vi "Save Output Settings to CSV.vi"(0 "time stamp":timestamp, 1 "Event Name":cluster{"string":string, string}, 2 "Modulatin Depth Sweep Parameters":T1={"f (Hz)"=200.0, "Number of steps"=2, "Total time (s)"=2.0, "Amplitude (V)"=1.0, "depth_start (0.0 %)"=50.0, "Channel (1:Channel 1)"=2, "fc (Hz)"=2000.0, "DC Offset (V)"=0.0, "depth_end (0.0 %)"=50.0} {"depth_end (0.0 %)" min=0.0 max=120.0 format="%.1f"; "DC Offset (V)" min=-20.0 max=20.0 format="%#_13g"; "fc (Hz)" min=0.0; "Channel (1:Channel 1)" items=["Channel 1"=1, "Channel 2"=2]; "depth_start (0.0 %)" min=0.0 max=120.0 format="%.1f"; "Amplitude (V)" min=0.0 max=20.0 format="%#_13g"; "Total time (s)" min=0.0; "Number of steps" min=2; "f (Hz)" min=0.0}, 3 "File numbers":i32[](array[numeric]), 4 "File Parameters":cluster{"Path":path, "Recording Name":string}={"Path"=path "D:/data/Lucas/20210707_lucas_test_saving", "Recording Name"=""}, 5 "error in (no error)":errorcluster, 6 "Output Parameters":T6={"Signal Parameters"={"P2P Amplitude (V)"=3.0, "Frequency (Hz)"=100000.0, "DC Offset ( V)"=0.0, "Waveform Function (0: Sine)"=0}, "Modulation Parameters"={"Waveform"=0, "Frequency (Hz)"=1000.0, "Depth (%)"=0.0, "Type"=100}} {"Modulation Parameters"."Type" items=["Amplitude", "Frequency"]; "Modulation Parameters"."Depth (%)" min=0.0 max=100.0 format="%.1f"; "Modulation Parameters"."Waveform" items=["Sine", "Square", "Triangle", "UpRamp", "DnRamp", "Noise", "Arb"]; "Signal Parameters"."Waveform Function (0: Sine)" items=["Sine", "Square", "Triangle", "DC", "Pulse", "Arb"]; "Signal Parameters"."P2P Amplitude (V)" min=0.0 max=20.0}, 7 "DIO":T5, 8 "Frequency Sweep I Parameters":T4={"f_start (Hz)"=0.0, "f_end (Hz)"=0.0, "Number of steps"=2, "Total time (s)"=0.0, "fc (Hz)"=2000.0, "Modulation Depth (0.0 %)"=0.0, "Channel (1:Channel 1)"=1, "amp (V)"=1.0, "DC Offset (V)"=0.0} {"DC Offset (V)" min=-20.0 max=20.0 format="%#_13g"; "amp (V)" min=0.0 max=20.0 format="%#_13g"; "Channel (1:Channel 1)" items=["Channel 1"=1, "Channel 2"=2]; "Modulation Depth (0.0 %)" min=0.0 max=120.0 format="%.1f"; "fc (Hz)" min=0.0 format="%#_13g"; "Total time (s)" min=0.0; "Number of steps" min=2; "f_end (Hz)" min=0.0; "f_start (Hz)" min=0.0}, 9 "Channel output":bool, 10 "Frequency Sweep II Parameters":T3={"f (Hz)"=0.0, "Number of steps"=2, "Total time (s)"=0.0, "fc_start (Hz)"=2000.0, "Modulation Depth (0.0 %)"=0.0, "Channel (1:Channel 1)"=1, "fc_end (Hz)"=2000.0, "amp (V)"=1.0, "DC Offset (V)"=0.0} {"DC Offset (V)" min=-20.0 max=20.0 format="%#_13g"; "amp (V)" min=0.0 max=20.0 format="%#_13g"; "fc_end (Hz)" min=0.0 format="%#_13g"; "Channel (1:Channel 1)" items=["Channel 1"=1, "Channel 2"=2]; "Modulation Depth (0.0 %)" min=0.0 max=120.0 format="%.1f"; "fc_start (Hz)" min=0.0 format="%#_13g"; "Total time (s)" min=0.0; "Number of steps" min=2; "f (Hz)" min=0.0}, 11 "Channel Modulation":bool, 12 "Amplitude Sweep Parameters":T2={"f (Hz)"=0.0, "Number of steps"=2, "Total time (s)"=0.0, "amp_start (V)"=2000.0, "Modulation Depth (0.0 %)"=0.0, "Channel (1:Channel 1)"=2, "amp_end (V)"=2000.0, "fc (Hz)"=0.0, "DC Offset (V)"=0.0} {"DC Offset (V)" min=-20.0 max=20.0 format="%#_13g"; "fc (Hz)" min=0.0; "amp_end (V)" min=0.0 max=20.0 format="%#_13g"; "Channel (1:Channel 1)" items=["Channel 1"=1, "Channel 2"=2]; "Modulation Depth (0.0 %)" min=0.0 max=120.0 format="%.1f"; "amp_start (V)" min=0.0 max=20.0 format="%#_13g"; "Total time (s)" min=0.0; "Number of steps" min=2; "f (Hz)" min=0.0}, 13 "Threshold Value":u32, 16 "Precheck duration":u32, 17 "Scenario Duration":u32, 18 "Release Duration":u32) -> (14 "output filename":string, 19 "error out":errorcluster)   [LabVIEW 2024]
uses:
  Type Definitions/Channel Parameters.ctl
  Type Definitions/Modulation Types.ctl
  RT Core/Type Definitions/DIO_Cluster.ctl
  Type Definitions/Frequency_sweep_I Parameters.ctl
  Type Definitions/Frequency_sweep_II Parameters.ctl
  Type Definitions/Amplitude_sweep Parameters.ctl
  Type Definitions/Depth_sweep Parameters.ctl
  <vilib>/Utility/file.llb/Write Delimited Spreadsheet (string).vi
panel:
  out "Array":string[](array[string])
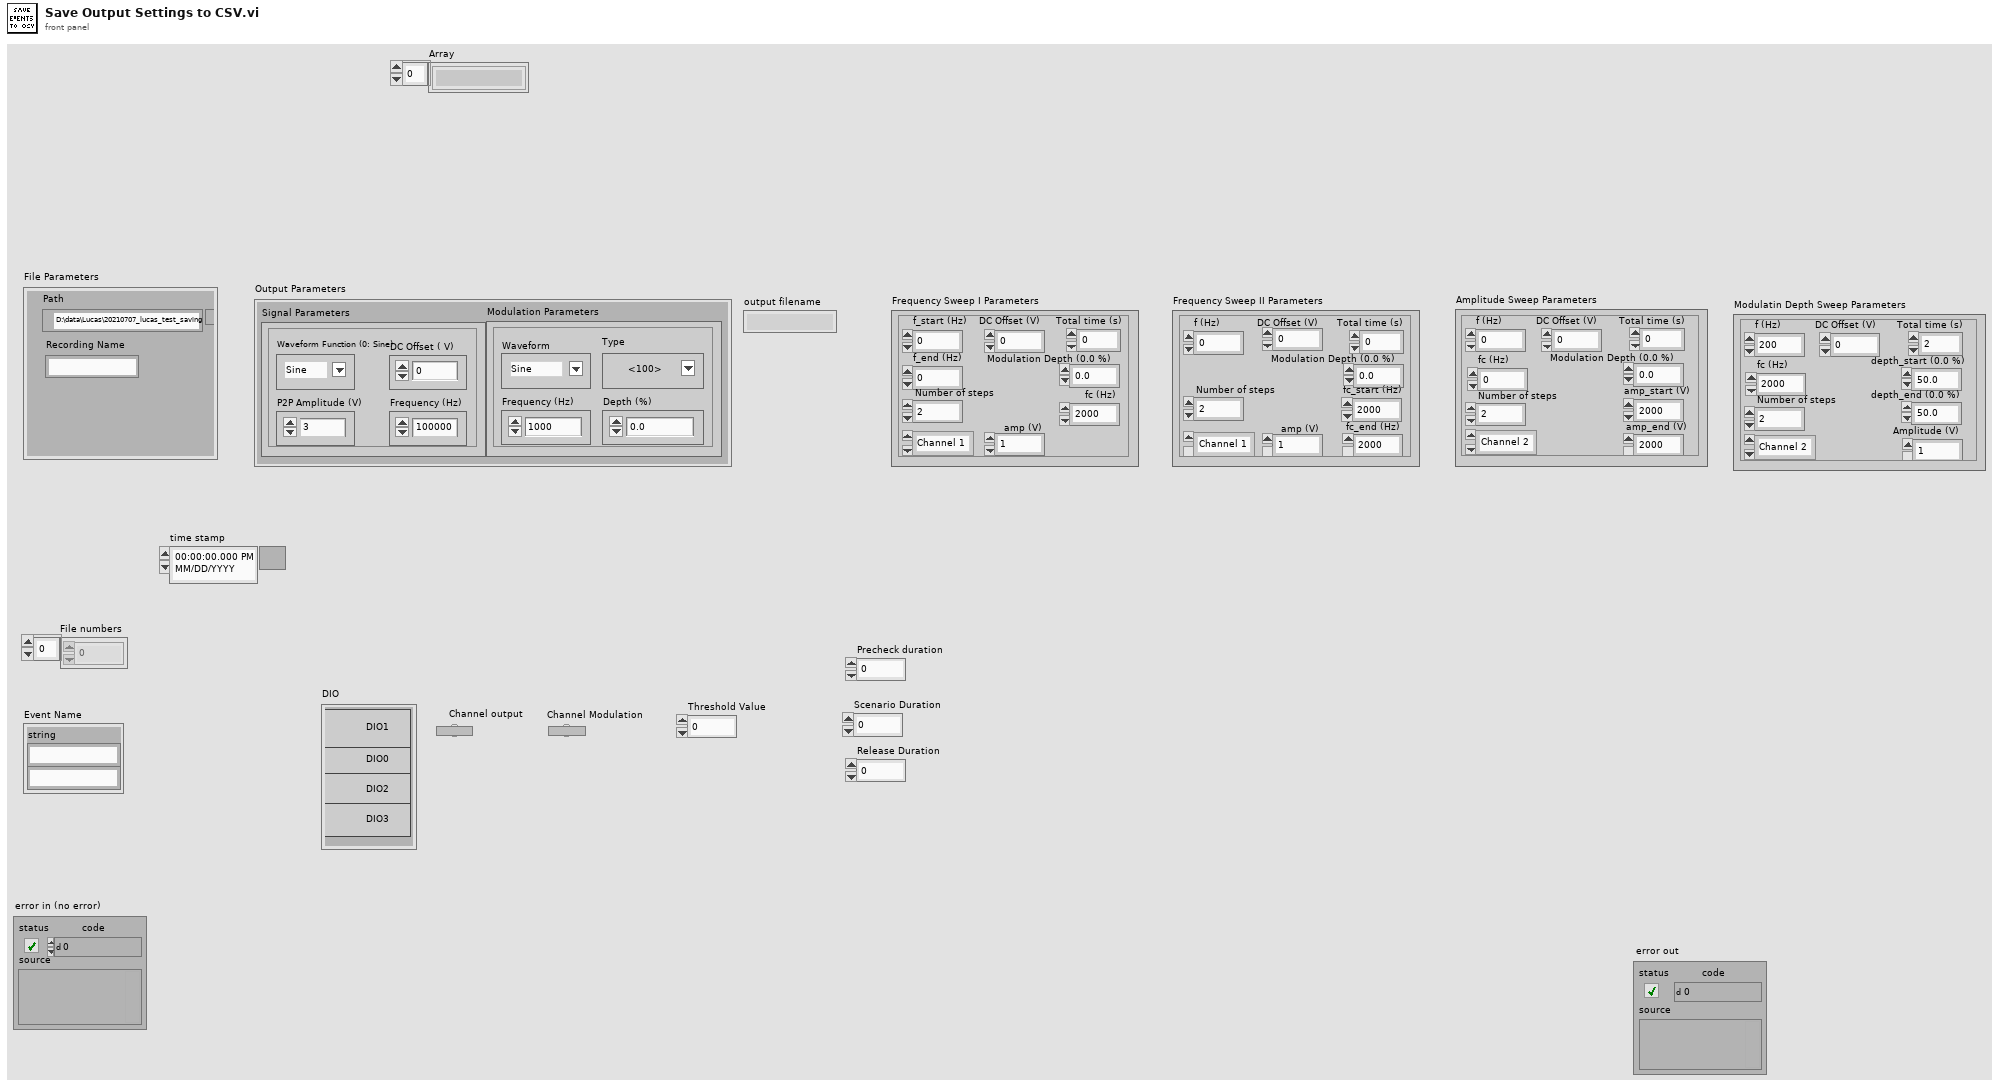
[diagram p1: front panel]
types:
  T1 = typedef "Depth_sweep Parameters.ctl" = cluster{"f (Hz)":dbl, "Number of steps":i32, "Total time (s)":dbl, "Amplitude (V)":dbl, "depth_start (0.0 %)":dbl, "Channel (1:Channel 1)":i32, "fc (Hz)":dbl, "DC Offset (V)":dbl, "depth_end (0.0 %)":dbl}
  T2 = typedef "Amplitude_sweep Parameters.ctl" = cluster{"f (Hz)":dbl, "Number of steps":i32, "Total time (s)":dbl, "amp_start (V)":dbl, "Modulation Depth (0.0 %)":dbl, "Channel (1:Channel 1)":i32, "amp_end (V)":dbl, "fc (Hz)":dbl, "DC Offset (V)":dbl}
  T3 = typedef "Frequency_sweep_II Parameters.ctl" = cluster{"f (Hz)":dbl, "Number of steps":i32, "Total time (s)":dbl, "fc_start (Hz)":dbl, "Modulation Depth (0.0 %)":dbl, "Channel (1:Channel 1)":i32, "fc_end (Hz)":dbl, "amp (V)":dbl, "DC Offset (V)":dbl}
  T4 = typedef "Frequency_sweep_I Parameters.ctl" = cluster{"f_start (Hz)":dbl, "f_end (Hz)":dbl, "Number of steps":i32, "Total time (s)":dbl, "fc (Hz)":dbl, "Modulation Depth (0.0 %)":dbl, "Channel (1:Channel 1)":i32, "amp (V)":dbl, "DC Offset (V)":dbl}
  T5 = typedef "DIO_Cluster.ctl" = cluster{"DIO0":bool, "DIO1":bool, "DIO2":bool, "DIO3":bool}
  T6 = typedef "Channel Parameters.ctl" = cluster{"Signal Parameters":cluster{"P2P Amplitude (V)":dbl, "Frequency (Hz)":dbl, "DC Offset ( V)":dbl, "Waveform Function (0: Sine)":u16}, "Modulation Parameters":cluster{"Waveform":u16, "Frequency (Hz)":dbl, "Depth (%)":dbl, "Type":T7}}
  T7 = typedef "Modulation Types.ctl" = u16
  T8 = cluster{"P2P Amplitude (V)":dbl, "Frequency (Hz)":dbl, "DC Offset ( V)":dbl, "Waveform Function (0: Sine)":u16}
  T9 = cluster{"Waveform":u16, "Frequency (Hz)":dbl, "Depth (%)":dbl, "Type":T7}
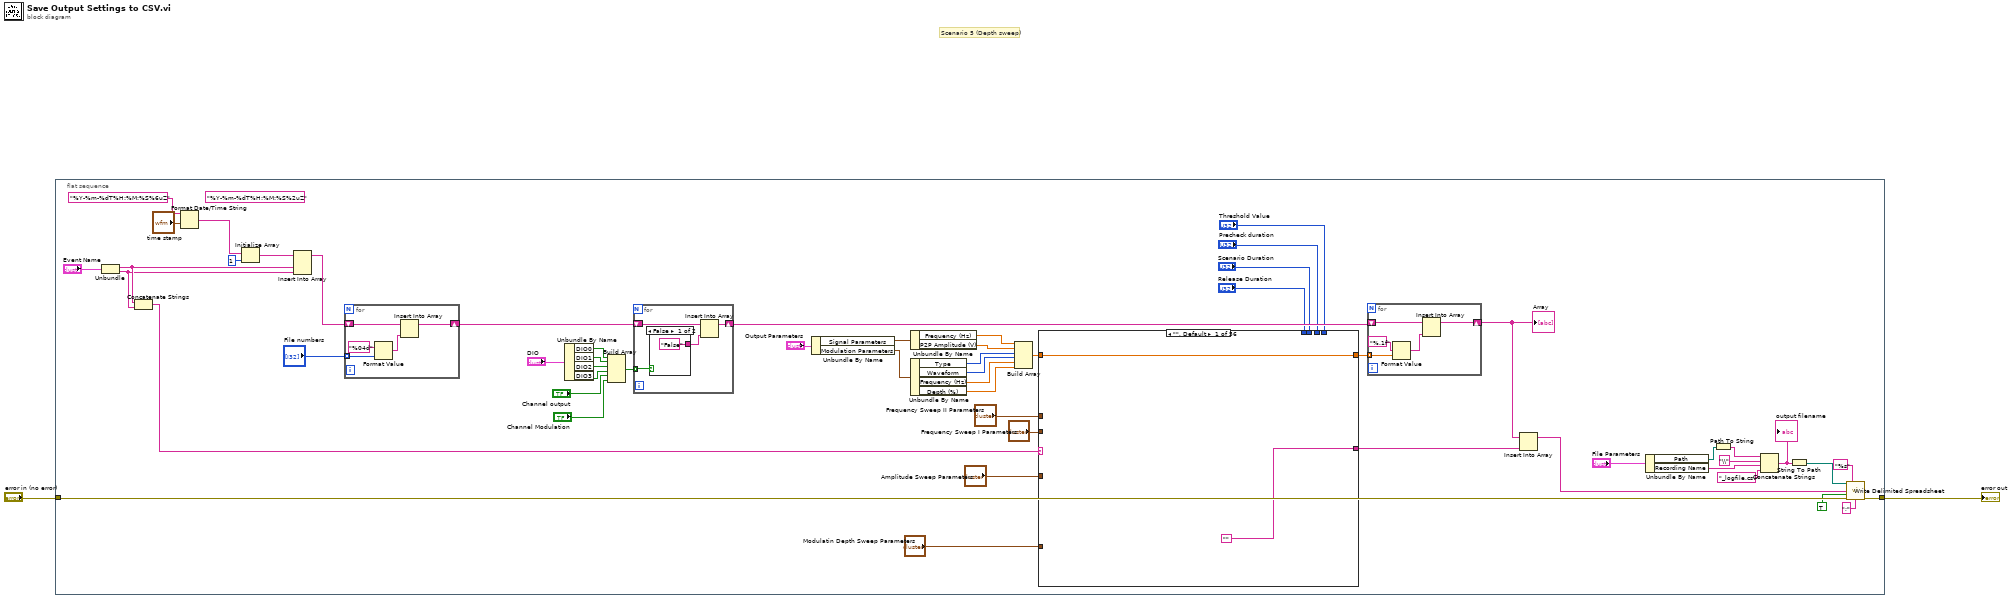
[diagram p0: block diagram]
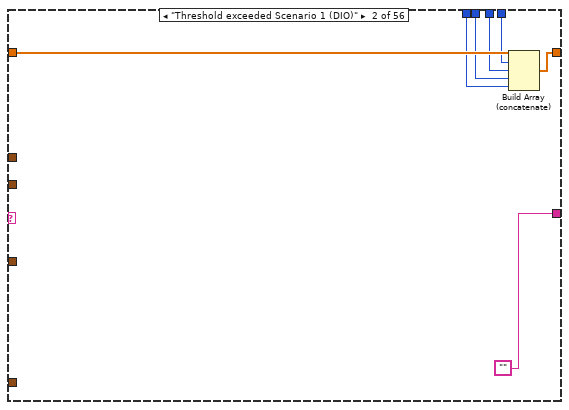
[diagram p2: hidden frame]
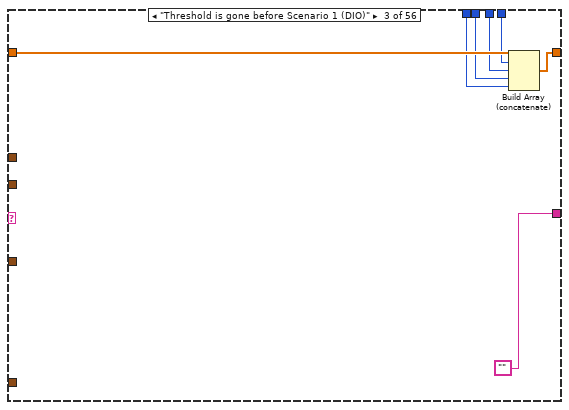
[diagram p3: hidden frame]
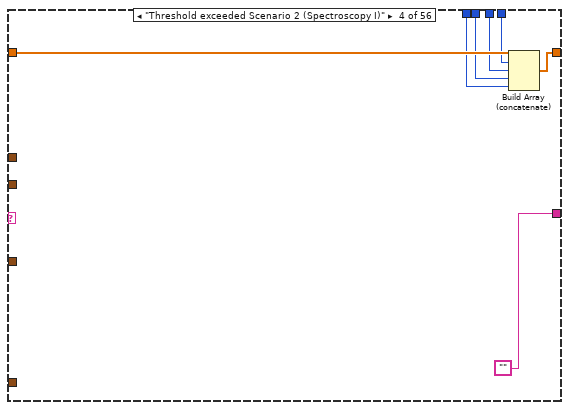
[diagram p4: hidden frame]
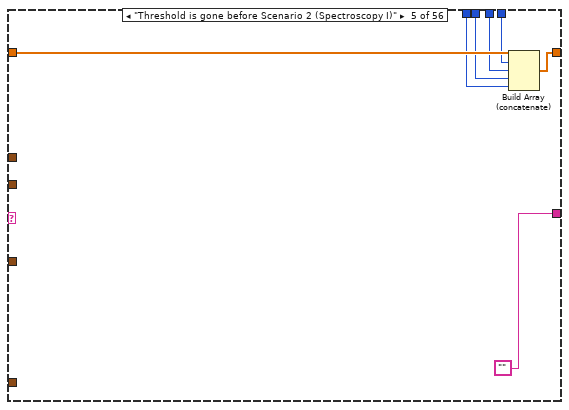
[diagram p5: hidden frame]
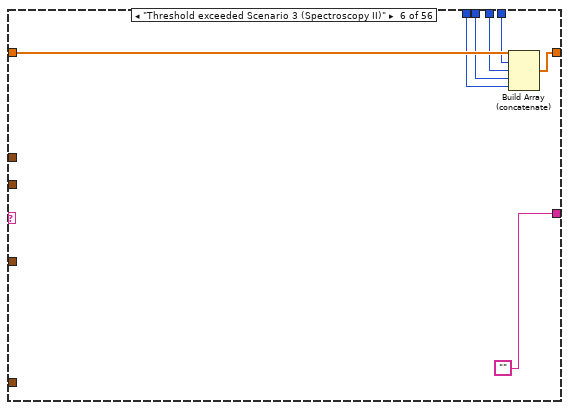
[diagram p6: hidden frame]
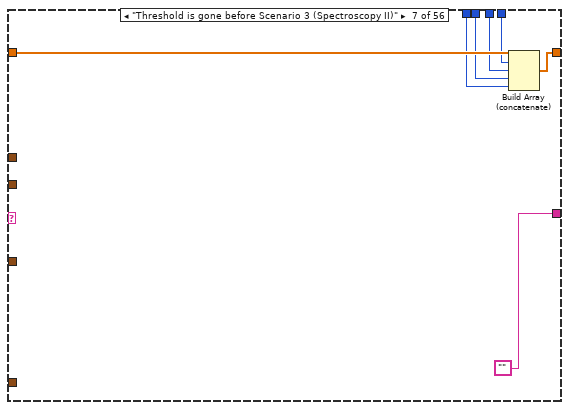
[diagram p7: hidden frame]
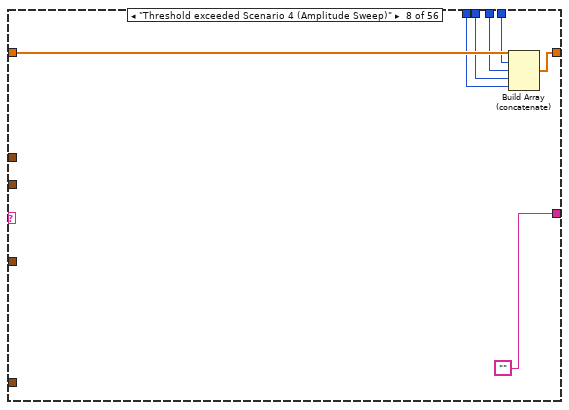
[diagram p8: hidden frame]
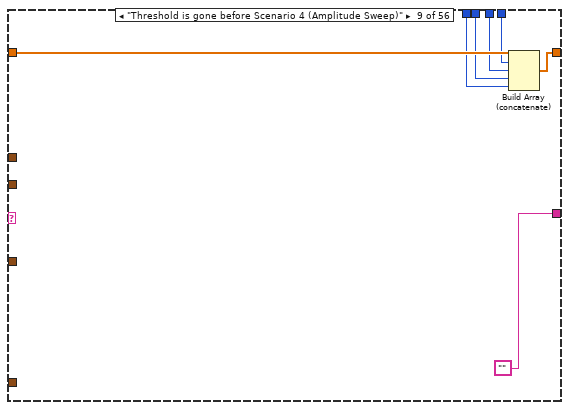
[diagram p9: hidden frame]
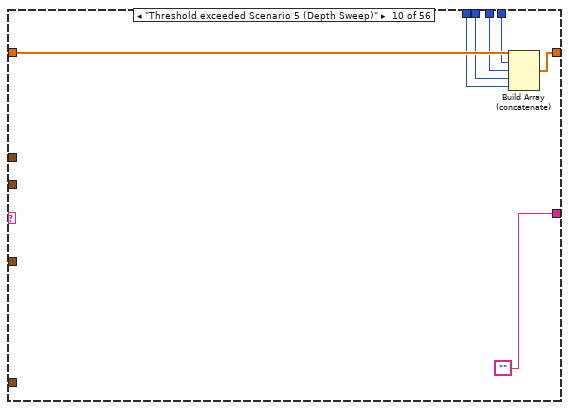
[diagram p10: hidden frame]
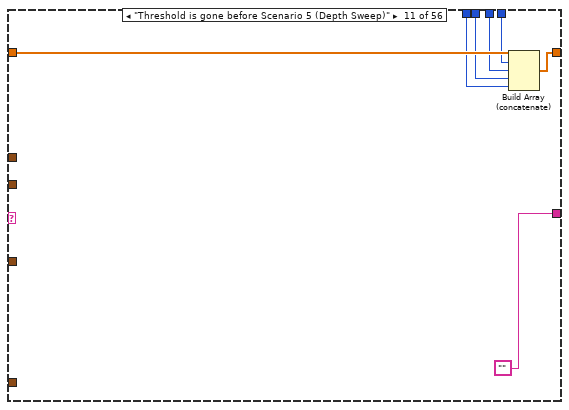
[diagram p11: hidden frame]
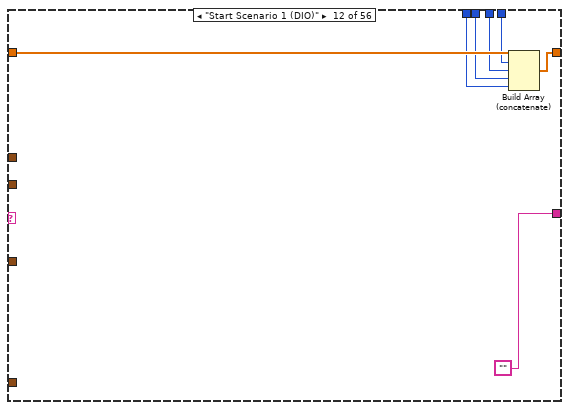
[diagram p12: hidden frame]
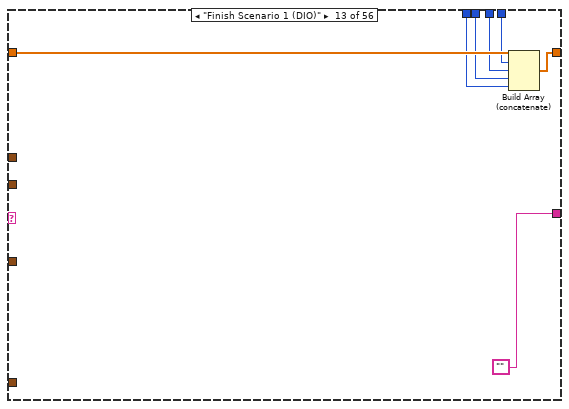
[diagram p13: hidden frame]
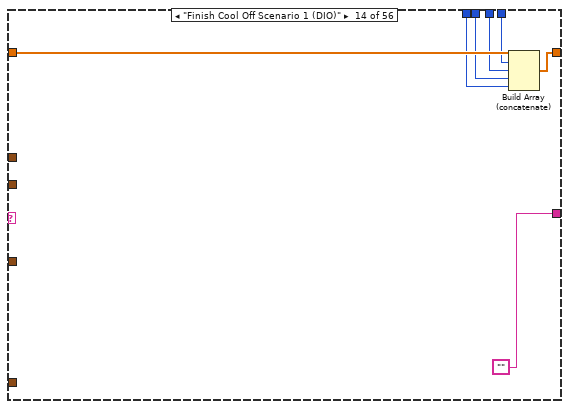
[diagram p14: hidden frame]
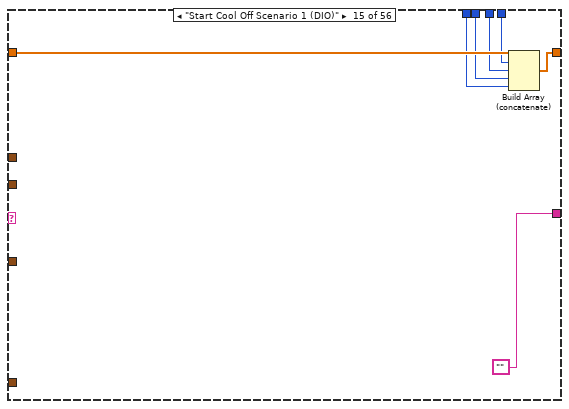
[diagram p15: hidden frame]
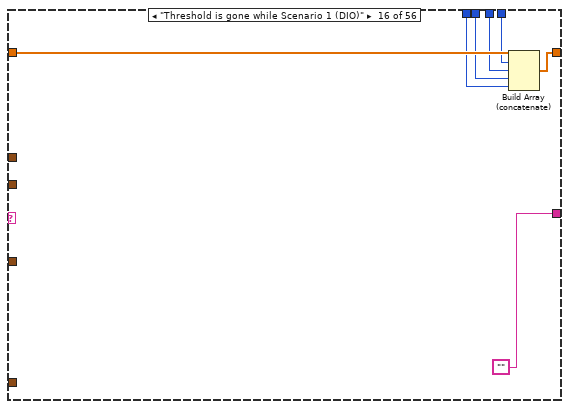
[diagram p16: hidden frame]
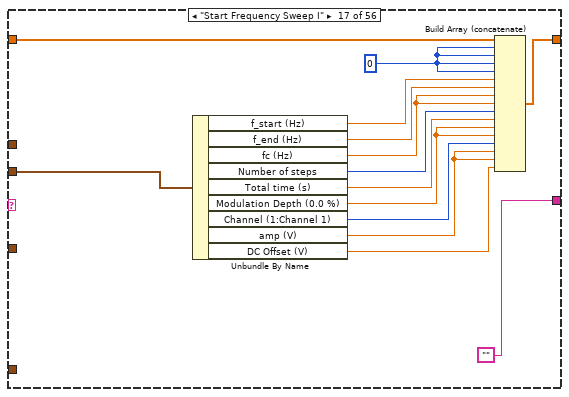
[diagram p17: hidden frame]
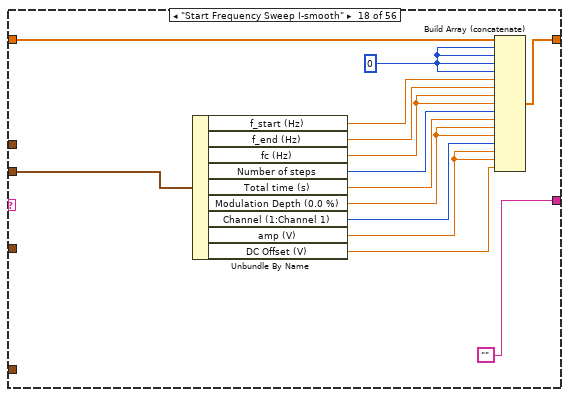
[diagram p18: hidden frame]
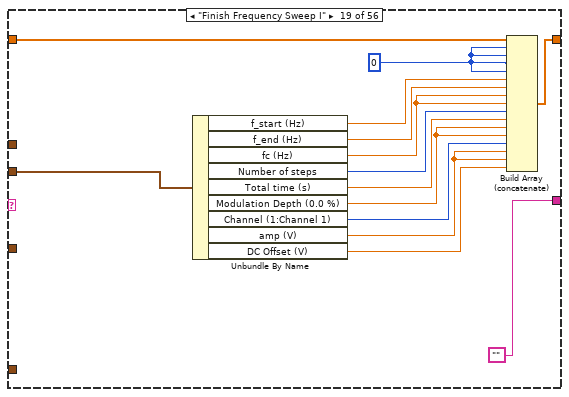
[diagram p19: hidden frame]
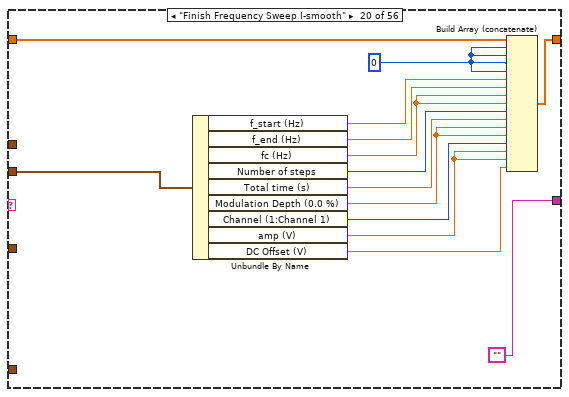
[diagram p20: hidden frame]
diagram:
  # "Scenario 5 (Depth sweep)"
  n1 = flat-sequence {
    tunnel: [w47] -> w1
    tunnel: "error in (no error)" -> [w58]
    frame #0 {
      (unwired) "%Y-%m-%dT%H:%M:%S%2uZ" ("time format string (%c)")
      n2 = Unbundle("Event Name") -> ("string"=w5:string, w4:string)
      n3 = Concatenate Strings(w5, w4) -> (w7:string)
      n4 = Format Date/Time String(time format string (%c)="%Y-%m-%dT%H:%M:%S%6uZ", seconds (now)="time stamp") -> (date/time string=w8:string)  [unwired: 1 in]
      n5 = Initialize Array "Initialize Array"(w8, 1 ("dimension size")) -> (w31:string[])
      n6 = Insert Into Array "Insert Into Array"(array=w31, new element #1=w5, new element #2=w4) -> (w30:string[])  [unwired: 1 in]
      n7 = for {
        tunnel: "File numbers" -> [w788] mode=indexing
        shift-right: [w790] -> w28
        shift-left: w30 -> [w789]
        n8 = Format Value(format string="%04d", value (0)=w788) -> (output string=w786:string)  [unwired: 1 in]
        n9 = Insert Into Array "Insert Into Array"(array=w789, new element=w786) -> (w790:string[])  [unwired: 1 in]
      }
      n10 = Unbundle By Name("DIO") -> ("DIO0"=w41:bool, "DIO1"=w40:bool, "DIO2"=w43:bool, "DIO3"=w44:bool)
      n11 = Build Array(w41, w40, w43, w44, "Channel output", "Channel Modulation") -> (w42:bool[])
      n12 = for {
        tunnel: w42 -> [w798] mode=indexing
        shift-right: [w796] -> w27
        shift-left: w28 -> [w797]
        n13 = case shown="False" w798 {
          tunnel: ["False" "True"] -> w799
          frame False {
          }
          frame True {
          }
        }
        n14 = Insert Into Array(array=w797, new element=w799) -> (w796:string[])  [unwired: 1 in]
      }
      n15 = Unbundle By Name("Output Parameters") -> ("Signal Parameters"=w34:T8, "Modulation Parameters"=w33:T9)
      n16 = Unbundle By Name(w33) -> ("Type"=w24:T7, "Waveform"=w38:u16, "Frequency (Hz)"=w37:dbl, "Depth (%)"=w39:dbl)
      n17 = Unbundle By Name(w34) -> ("Frequency (Hz)"=w25:dbl, "P2P Amplitude (V)"=w36:dbl)
      n18 = Build Array(w25, w36, w24, w38, w37, w39) -> (w23:dbl[])
      n19 = case shown="\"\", Default" w7 {
        tunnel: w23 -> [w60 w67 w74 w81 w88 w95 w102 w109 w116 w123 w130 w137 w144 w151 w158 w165 w179 w193 w207 w221 w235 w244 w269 w286 w303 w320 w334 w348 w362 w376 w390 w407 w424 w441 w458 w475 w489 w503 w517 w531 w545 w562 w579 w596 w613 w630 w644 w658 w672 w686 w700 w717 w734 w751 w768 w785]
        tunnel: [w60 w63 w70 w77 w84 w91 w98 w105 w112 w119 w126 w133 w140 w147 w154 w161 w178 w192 w206 w220 w234 w252 w268 w285 w302 w319 w333 w347 w361 w375 w389 w406 w423 w440 w457 w474 w488 w502 w516 w530 w544 w561 w578 w595 w612 w629 w643 w657 w671 w685 w699 w716 w733 w750 w767 w784] -> w22
        tunnel: "Frequency Sweep I Parameters" -> [_ _ _ _ _ _ _ _ _ _ _ _ _ _ _ _ w171 w185 w199 w213 w227 w245 w261 w278 w295 w312 _ _ _ _ _ _ _ _ _ _ _ _ _ _ _ _ _ _ _ _ _ _ _ _ _ _ _ _ _ _]
        tunnel: "Frequency Sweep II Parameters" -> [_ _ _ _ _ _ _ _ _ _ _ _ _ _ _ _ _ _ _ _ _ _ _ _ _ _ w326 w340 w354 w368 w382 w399 w416 w433 w450 w467 _ _ _ _ _ _ _ _ _ _ _ _ _ _ _ _ _ _ _ _]
        tunnel: "Threshold Value" -> [_ w66 w73 w80 w87 w94 w101 w108 w115 w122 w129 w136 w143 w150 w157 w164 _ _ _ _ _ w243 w260 w277 w294 w311 _ _ _ _ _ w398 w415 w432 w449 w466 _ _ _ _ _ w552 w569 w586 w603 w620 _ _ _ _ _ w701 w718 w735 w752 w769]
        tunnel: "Scenario Duration" -> [_ w65 w72 w79 w86 w93 w100 w107 w114 w121 w128 w135 w142 w149 w156 w163 _ _ _ _ _ w242 w259 w276 w293 w310 _ _ _ _ _ w397 w414 w431 w448 w465 _ _ _ _ _ w551 w568 w585 w602 w619 _ _ _ _ _ w703 w720 w737 w754 w771]
        tunnel: "Release Duration" -> [_ w64 w71 w78 w85 w92 w99 w106 w113 w120 w127 w134 w141 w148 w155 w162 _ _ _ _ _ w241 w258 w275 w292 w309 _ _ _ _ _ w396 w413 w430 w447 w464 _ _ _ _ _ w550 w567 w584 w601 w618 _ _ _ _ _ w704 w721 w738 w755 w772]
        tunnel: "Amplitude Sweep Parameters" -> [_ _ _ _ _ _ _ _ _ _ _ _ _ _ _ _ _ _ _ _ _ _ _ _ _ _ _ _ _ _ _ _ _ _ _ _ w487 w501 w515 w529 w543 w560 w577 w594 w611 w628 _ _ _ _ _ _ _ _ _ _]
        tunnel: ["" "" "" "" "" "" "" "" "" "" "" "" "" "" "" "" "" "" "" "" "" "" "" "" "" "" "" "" "" "" "" "" "" "" "" "" "" "" "" "" "" "" "" "" "" "" "" "" "" "" "" "" "" "" "" ""] -> w12
        tunnel: "Precheck duration" -> [_ w61 w68 w75 w82 w89 w96 w103 w110 w117 w124 w131 w138 w145 w152 w159 _ _ _ _ _ w237 w254 w271 w288 w305 _ _ _ _ _ w392 w409 w426 w443 w460 _ _ _ _ _ w547 w564 w581 w598 w615 _ _ _ _ _ w702 w719 w736 w753 w770]
        tunnel: "Modulatin Depth Sweep Parameters" -> [_ _ _ _ _ _ _ _ _ _ _ _ _ _ _ _ _ _ _ _ _ _ _ _ _ _ _ _ _ _ _ _ _ _ _ _ _ _ _ _ _ _ _ _ _ _ w640 w654 w668 w682 w696 w714 w731 w748 w765 w782]
        frame "", Default {
        }
        frame "Threshold exceeded Scenario 1 (DIO)" {
          n20 = Build Array (concatenate)(w67, w66, w61, w65, w64) -> (w63:dbl[])
        }
        frame "Threshold is gone before Scenario 1 (DIO)" {
          n21 = Build Array (concatenate)(w74, w73, w68, w72, w71) -> (w70:dbl[])
        }
        frame "Threshold exceeded Scenario 2 (Spectroscopy I)" {
          n22 = Build Array (concatenate)(w81, w80, w75, w79, w78) -> (w77:dbl[])
        }
        frame "Threshold is gone before Scenario 2 (Spectroscopy I)" {
          n23 = Build Array (concatenate)(w88, w87, w82, w86, w85) -> (w84:dbl[])
        }
        frame "Threshold exceeded Scenario 3 (Spectroscopy II)" {
          n24 = Build Array (concatenate)(w95, w94, w89, w93, w92) -> (w91:dbl[])
        }
        frame "Threshold is gone before Scenario 3 (Spectroscopy II)" {
          n25 = Build Array (concatenate)(w102, w101, w96, w100, w99) -> (w98:dbl[])
        }
        frame "Threshold exceeded Scenario 4 (Amplitude Sweep)" {
          n26 = Build Array (concatenate)(w109, w108, w103, w107, w106) -> (w105:dbl[])
        }
        frame "Threshold is gone before Scenario 4 (Amplitude Sweep)" {
          n27 = Build Array (concatenate)(w116, w115, w110, w114, w113) -> (w112:dbl[])
        }
        frame "Threshold exceeded Scenario 5 (Depth Sweep)" {
          n28 = Build Array (concatenate)(w123, w122, w117, w121, w120) -> (w119:dbl[])
        }
        frame "Threshold is gone before Scenario 5 (Depth Sweep)" {
          n29 = Build Array (concatenate)(w130, w129, w124, w128, w127) -> (w126:dbl[])
        }
        frame "Start Scenario 1 (DIO)" {
          n30 = Build Array (concatenate)(w137, w136, w131, w135, w134) -> (w133:dbl[])
        }
        frame "Finish Scenario 1 (DIO)" {
          n31 = Build Array (concatenate)(w144, w143, w138, w142, w141) -> (w140:dbl[])
        }
        frame "Finish Cool Off Scenario 1 (DIO)" {
          n32 = Build Array (concatenate)(w151, w150, w145, w149, w148) -> (w147:dbl[])
        }
        frame "Start Cool Off Scenario 1 (DIO)" {
          n33 = Build Array (concatenate)(w158, w157, w152, w156, w155) -> (w154:dbl[])
        }
        frame "Threshold is gone while Scenario 1 (DIO)" {
          n34 = Build Array (concatenate)(w165, w164, w159, w163, w162) -> (w161:dbl[])
        }
        frame "Start Frequency Sweep I" {
          w167 = 0
          n35 = Unbundle By Name(w171) -> ("f_start (Hz)"=w177:dbl, "f_end (Hz)"=w176:dbl, "fc (Hz)"=w175:dbl, "Number of steps"=w174:i32, "Total time (s)"=w173:dbl, "Modulation Depth (0.0 %)"=w166:dbl, "Channel (1:Channel 1)"=w172:i32, "amp (V)"=w169:dbl, "DC Offset (V)"=w168:dbl)
          n36 = Build Array (concatenate)(w179, w167, w167, w167, w167, w177, w176, w175, w175, w174, w173, w166, w166, w172, w169, w169, w168) -> (w178:dbl[])
        }
        frame "Start Frequency Sweep I-smooth" {
          w181 = 0
          n37 = Unbundle By Name(w185) -> ("f_start (Hz)"=w191:dbl, "f_end (Hz)"=w190:dbl, "fc (Hz)"=w189:dbl, "Number of steps"=w188:i32, "Total time (s)"=w187:dbl, "Modulation Depth (0.0 %)"=w180:dbl, "Channel (1:Channel 1)"=w186:i32, "amp (V)"=w183:dbl, "DC Offset (V)"=w182:dbl)
          n38 = Build Array (concatenate)(w193, w181, w181, w181, w181, w191, w190, w189, w189, w188, w187, w180, w180, w186, w183, w183, w182) -> (w192:dbl[])
        }
        frame "Finish Frequency Sweep I" {
          w195 = 0
          n39 = Unbundle By Name(w199) -> ("f_start (Hz)"=w205:dbl, "f_end (Hz)"=w204:dbl, "fc (Hz)"=w203:dbl, "Number of steps"=w202:i32, "Total time (s)"=w201:dbl, "Modulation Depth (0.0 %)"=w194:dbl, "Channel (1:Channel 1)"=w200:i32, "amp (V)"=w197:dbl, "DC Offset (V)"=w196:dbl)
          n40 = Build Array (concatenate)(w207, w195, w195, w195, w195, w205, w204, w203, w203, w202, w201, w194, w194, w200, w197, w197, w196) -> (w206:dbl[])
        }
        frame "Finish Frequency Sweep I-smooth" {
          w209 = 0
          n41 = Unbundle By Name(w213) -> ("f_start (Hz)"=w219:dbl, "f_end (Hz)"=w218:dbl, "fc (Hz)"=w217:dbl, "Number of steps"=w216:i32, "Total time (s)"=w215:dbl, "Modulation Depth (0.0 %)"=w208:dbl, "Channel (1:Channel 1)"=w214:i32, "amp (V)"=w211:dbl, "DC Offset (V)"=w210:dbl)
          n42 = Build Array (concatenate)(w221, w209, w209, w209, w209, w219, w218, w217, w217, w216, w215, w208, w208, w214, w211, w211, w210) -> (w220:dbl[])
        }
        frame "Sweep Parameters I Change" {
          w223 = 0
          n43 = Unbundle By Name(w227) -> ("f_start (Hz)"=w233:dbl, "f_end (Hz)"=w232:dbl, "fc (Hz)"=w231:dbl, "Number of steps"=w230:i32, "Total time (s)"=w229:dbl, "Modulation Depth (0.0 %)"=w222:dbl, "Channel (1:Channel 1)"=w228:i32, "amp (V)"=w225:dbl, "DC Offset (V)"=w224:dbl)
          n44 = Build Array (concatenate)(w235, w223, w223, w223, w223, w233, w232, w231, w231, w230, w229, w222, w222, w228, w225, w225, w224) -> (w234:dbl[])
        }
        frame "Start Scenario 2 (Spectroscopy I)" {
          n45 = Unbundle By Name(w245) -> ("f_start (Hz)"=w251:dbl, "f_end (Hz)"=w250:dbl, "fc (Hz)"=w249:dbl, "Number of steps"=w248:i32, "Total time (s)"=w247:dbl, "Modulation Depth (0.0 %)"=w236:dbl, "Channel (1:Channel 1)"=w246:i32, "amp (V)"=w239:dbl, "DC Offset (V)"=w238:dbl)
          n46 = Build Array (concatenate)(w244, w243, w237, w242, w241, w251, w250, w249, w249, w248, w247, w236, w236, w246, w239, w239, w238) -> (w252:dbl[])
        }
        frame "Finish Scenario 2 (Spectroscopy I)" {
          n47 = Unbundle By Name(w261) -> ("f_start (Hz)"=w267:dbl, "f_end (Hz)"=w266:dbl, "fc (Hz)"=w265:dbl, "Number of steps"=w264:i32, "Total time (s)"=w263:dbl, "Modulation Depth (0.0 %)"=w253:dbl, "Channel (1:Channel 1)"=w262:i32, "amp (V)"=w256:dbl, "DC Offset (V)"=w255:dbl)
          n48 = Build Array (concatenate)(w269, w260, w254, w259, w258, w267, w266, w265, w265, w264, w263, w253, w253, w262, w256, w256, w255) -> (w268:dbl[])
        }
        frame "Finish Cool Off Scenario 2 (Spectroscopy I)" {
          n49 = Unbundle By Name(w278) -> ("f_start (Hz)"=w284:dbl, "f_end (Hz)"=w283:dbl, "fc (Hz)"=w282:dbl, "Number of steps"=w281:i32, "Total time (s)"=w280:dbl, "Modulation Depth (0.0 %)"=w270:dbl, "Channel (1:Channel 1)"=w279:i32, "amp (V)"=w273:dbl, "DC Offset (V)"=w272:dbl)
          n50 = Build Array (concatenate)(w286, w277, w271, w276, w275, w284, w283, w282, w282, w281, w280, w270, w270, w279, w273, w273, w272) -> (w285:dbl[])
        }
        frame "Start Cool Off Scenario 2 (Spectroscopy I)" {
          n51 = Unbundle By Name(w295) -> ("f_start (Hz)"=w301:dbl, "f_end (Hz)"=w300:dbl, "fc (Hz)"=w299:dbl, "Number of steps"=w298:i32, "Total time (s)"=w297:dbl, "Modulation Depth (0.0 %)"=w287:dbl, "Channel (1:Channel 1)"=w296:i32, "amp (V)"=w290:dbl, "DC Offset (V)"=w289:dbl)
          n52 = Build Array (concatenate)(w303, w294, w288, w293, w292, w301, w300, w299, w299, w298, w297, w287, w287, w296, w290, w290, w289) -> (w302:dbl[])
        }
        frame "Threshold is gone while Scenario 2 (Spectroscopy I)" {
          n53 = Unbundle By Name(w312) -> ("f_start (Hz)"=w318:dbl, "f_end (Hz)"=w317:dbl, "fc (Hz)"=w316:dbl, "Number of steps"=w315:i32, "Total time (s)"=w314:dbl, "Modulation Depth (0.0 %)"=w304:dbl, "Channel (1:Channel 1)"=w313:i32, "amp (V)"=w307:dbl, "DC Offset (V)"=w306:dbl)
          n54 = Build Array (concatenate)(w320, w311, w305, w310, w309, w318, w317, w316, w316, w315, w314, w304, w304, w313, w307, w307, w306) -> (w319:dbl[])
        }
        frame "Start Frequency Sweep II" {
          w322 = 0
          n55 = Unbundle By Name(w326) -> ("f (Hz)"=w332:dbl, "fc_start (Hz)"=w331:dbl, "fc_end (Hz)"=w330:dbl, "Number of steps"=w329:i32, "Total time (s)"=w328:dbl, "Modulation Depth (0.0 %)"=w321:dbl, "Channel (1:Channel 1)"=w327:i32, "amp (V)"=w324:dbl, "DC Offset (V)"=w323:dbl)
          n56 = Build Array (concatenate)(w334, w322, w322, w322, w322, w332, w332, w331, w330, w329, w328, w321, w321, w327, w324, w324, w323) -> (w333:dbl[])
        }
        frame "Start Frequency Sweep II-smooth" {
          w336 = 0
          n57 = Unbundle By Name(w340) -> ("f (Hz)"=w346:dbl, "fc_start (Hz)"=w345:dbl, "fc_end (Hz)"=w344:dbl, "Number of steps"=w343:i32, "Total time (s)"=w342:dbl, "Modulation Depth (0.0 %)"=w335:dbl, "Channel (1:Channel 1)"=w341:i32, "amp (V)"=w338:dbl, "DC Offset (V)"=w337:dbl)
          n58 = Build Array (concatenate)(w348, w336, w336, w336, w336, w346, w346, w345, w344, w343, w342, w335, w335, w341, w338, w338, w337) -> (w347:dbl[])
        }
        frame "Finish Frequency Sweep II" {
          w350 = 0
          n59 = Unbundle By Name(w354) -> ("f (Hz)"=w360:dbl, "fc_start (Hz)"=w359:dbl, "fc_end (Hz)"=w358:dbl, "Number of steps"=w357:i32, "Total time (s)"=w356:dbl, "Modulation Depth (0.0 %)"=w349:dbl, "Channel (1:Channel 1)"=w355:i32, "amp (V)"=w352:dbl, "DC Offset (V)"=w351:dbl)
          n60 = Build Array (concatenate)(w362, w350, w350, w350, w350, w360, w360, w359, w358, w357, w356, w349, w349, w355, w352, w352, w351) -> (w361:dbl[])
        }
        frame "Finish Frequency Sweep II-smooth" {
          w364 = 0
          n61 = Unbundle By Name(w368) -> ("f (Hz)"=w374:dbl, "fc_start (Hz)"=w373:dbl, "fc_end (Hz)"=w372:dbl, "Number of steps"=w371:i32, "Total time (s)"=w370:dbl, "Modulation Depth (0.0 %)"=w363:dbl, "Channel (1:Channel 1)"=w369:i32, "amp (V)"=w366:dbl, "DC Offset (V)"=w365:dbl)
          n62 = Build Array (concatenate)(w376, w364, w364, w364, w364, w374, w374, w373, w372, w371, w370, w363, w363, w369, w366, w366, w365) -> (w375:dbl[])
        }
        frame "Sweep Parameters II Change" {
          w378 = 0
          n63 = Unbundle By Name(w382) -> ("f (Hz)"=w388:dbl, "fc_start (Hz)"=w387:dbl, "fc_end (Hz)"=w386:dbl, "Number of steps"=w385:i32, "Total time (s)"=w384:dbl, "Modulation Depth (0.0 %)"=w377:dbl, "Channel (1:Channel 1)"=w383:i32, "amp (V)"=w380:dbl, "DC Offset (V)"=w379:dbl)
          n64 = Build Array (concatenate)(w390, w378, w378, w378, w378, w388, w388, w387, w386, w385, w384, w377, w377, w383, w380, w380, w379) -> (w389:dbl[])
        }
        frame "Start Scenario 3 (Spectroscopy II)" {
          n65 = Unbundle By Name(w399) -> ("f (Hz)"=w405:dbl, "fc_start (Hz)"=w404:dbl, "fc_end (Hz)"=w403:dbl, "Number of steps"=w402:i32, "Total time (s)"=w401:dbl, "Modulation Depth (0.0 %)"=w391:dbl, "Channel (1:Channel 1)"=w400:i32, "amp (V)"=w394:dbl, "DC Offset (V)"=w393:dbl)
          n66 = Build Array (concatenate)(w407, w398, w392, w397, w396, w405, w405, w404, w403, w402, w401, w391, w391, w400, w394, w394, w393) -> (w406:dbl[])
        }
        frame "Finish Scenario 3 (Spectroscopy II)" {
          n67 = Unbundle By Name(w416) -> ("f (Hz)"=w422:dbl, "fc_start (Hz)"=w421:dbl, "fc_end (Hz)"=w420:dbl, "Number of steps"=w419:i32, "Total time (s)"=w418:dbl, "Modulation Depth (0.0 %)"=w408:dbl, "Channel (1:Channel 1)"=w417:i32, "amp (V)"=w411:dbl, "DC Offset (V)"=w410:dbl)
          n68 = Build Array (concatenate)(w424, w415, w409, w414, w413, w422, w422, w421, w420, w419, w418, w408, w408, w417, w411, w411, w410) -> (w423:dbl[])
        }
        frame "Finish Cool Off Scenario 3 (Spectroscopy II)" {
          n69 = Unbundle By Name(w433) -> ("f (Hz)"=w439:dbl, "fc_start (Hz)"=w438:dbl, "fc_end (Hz)"=w437:dbl, "Number of steps"=w436:i32, "Total time (s)"=w435:dbl, "Modulation Depth (0.0 %)"=w425:dbl, "Channel (1:Channel 1)"=w434:i32, "amp (V)"=w428:dbl, "DC Offset (V)"=w427:dbl)
          n70 = Build Array (concatenate)(w441, w432, w426, w431, w430, w439, w439, w438, w437, w436, w435, w425, w425, w434, w428, w428, w427) -> (w440:dbl[])
        }
        frame "Start Cool Off Scenario 3 (Spectroscopy II)" {
          n71 = Unbundle By Name(w450) -> ("f (Hz)"=w456:dbl, "fc_start (Hz)"=w455:dbl, "fc_end (Hz)"=w454:dbl, "Number of steps"=w453:i32, "Total time (s)"=w452:dbl, "Modulation Depth (0.0 %)"=w442:dbl, "Channel (1:Channel 1)"=w451:i32, "amp (V)"=w445:dbl, "DC Offset (V)"=w444:dbl)
          n72 = Build Array (concatenate)(w458, w449, w443, w448, w447, w456, w456, w455, w454, w453, w452, w442, w442, w451, w445, w445, w444) -> (w457:dbl[])
        }
        frame "Threshold is gone while Scenario 3 (Spectroscopy II)" {
          n73 = Unbundle By Name(w467) -> ("f (Hz)"=w473:dbl, "fc_start (Hz)"=w472:dbl, "fc_end (Hz)"=w471:dbl, "Number of steps"=w470:i32, "Total time (s)"=w469:dbl, "Modulation Depth (0.0 %)"=w459:dbl, "Channel (1:Channel 1)"=w468:i32, "amp (V)"=w462:dbl, "DC Offset (V)"=w461:dbl)
          n74 = Build Array (concatenate)(w475, w466, w460, w465, w464, w473, w473, w472, w471, w470, w469, w459, w459, w468, w462, w462, w461) -> (w474:dbl[])
        }
        frame "Start Amplitude Sweep" {
          w477 = 0
          n75 = Unbundle By Name(w487) -> ("f (Hz)"=w486:dbl, "Number of steps"=w484:i32, "Total time (s)"=w483:dbl, "amp_start (V)"=w481:dbl, "Modulation Depth (0.0 %)"=w476:dbl, "Channel (1:Channel 1)"=w482:i32, "amp_end (V)"=w480:dbl, "fc (Hz)"=w485:dbl, "DC Offset (V)"=w478:dbl)
          n76 = Build Array (concatenate)(w489, w477, w477, w477, w477, w486, w486, w485, w485, w484, w483, w476, w476, w482, w481, w480, w478) -> (w488:dbl[])
        }
        frame "Start Amplitude Sweep-smooth" {
          w491 = 0
          n77 = Unbundle By Name(w501) -> ("f (Hz)"=w500:dbl, "Number of steps"=w498:i32, "Total time (s)"=w497:dbl, "amp_start (V)"=w495:dbl, "Modulation Depth (0.0 %)"=w490:dbl, "Channel (1:Channel 1)"=w496:i32, "amp_end (V)"=w494:dbl, "fc (Hz)"=w499:dbl, "DC Offset (V)"=w492:dbl)
          n78 = Build Array (concatenate)(w503, w491, w491, w491, w491, w500, w500, w499, w499, w498, w497, w490, w490, w496, w495, w494, w492) -> (w502:dbl[])
        }
        frame "Finish Amplitude Sweep" {
          w505 = 0
          n79 = Unbundle By Name(w515) -> ("f (Hz)"=w514:dbl, "Number of steps"=w512:i32, "Total time (s)"=w511:dbl, "amp_start (V)"=w509:dbl, "Modulation Depth (0.0 %)"=w504:dbl, "Channel (1:Channel 1)"=w510:i32, "amp_end (V)"=w508:dbl, "fc (Hz)"=w513:dbl, "DC Offset (V)"=w506:dbl)
          n80 = Build Array (concatenate)(w517, w505, w505, w505, w505, w514, w514, w513, w513, w512, w511, w504, w504, w510, w509, w508, w506) -> (w516:dbl[])
        }
        frame "Finish Amplitude Sweep-smooth" {
          w519 = 0
          n81 = Unbundle By Name(w529) -> ("f (Hz)"=w528:dbl, "Number of steps"=w526:i32, "Total time (s)"=w525:dbl, "amp_start (V)"=w523:dbl, "Modulation Depth (0.0 %)"=w518:dbl, "Channel (1:Channel 1)"=w524:i32, "amp_end (V)"=w522:dbl, "fc (Hz)"=w527:dbl, "DC Offset (V)"=w520:dbl)
          n82 = Build Array (concatenate)(w531, w519, w519, w519, w519, w528, w528, w527, w527, w526, w525, w518, w518, w524, w523, w522, w520) -> (w530:dbl[])
        }
        frame "Amplitude Sweep Parameters Change" {
          w533 = 0
          n83 = Unbundle By Name(w543) -> ("f (Hz)"=w542:dbl, "Number of steps"=w540:i32, "Total time (s)"=w539:dbl, "amp_start (V)"=w537:dbl, "Modulation Depth (0.0 %)"=w532:dbl, "Channel (1:Channel 1)"=w538:i32, "amp_end (V)"=w536:dbl, "fc (Hz)"=w541:dbl, "DC Offset (V)"=w534:dbl)
          n84 = Build Array (concatenate)(w545, w533, w533, w533, w533, w542, w542, w541, w541, w540, w539, w532, w532, w538, w537, w536, w534) -> (w544:dbl[])
        }
        frame "Start Scenario 4 (Amplitude Sweep)" {
          n85 = Unbundle By Name(w560) -> ("f (Hz)"=w559:dbl, "Number of steps"=w557:i32, "Total time (s)"=w556:dbl, "amp_start (V)"=w554:dbl, "Modulation Depth (0.0 %)"=w546:dbl, "Channel (1:Channel 1)"=w555:i32, "amp_end (V)"=w553:dbl, "fc (Hz)"=w558:dbl, "DC Offset (V)"=w548:dbl)
          n86 = Build Array (concatenate)(w562, w552, w547, w551, w550, w559, w559, w558, w558, w557, w556, w546, w546, w555, w554, w553, w548) -> (w561:dbl[])
        }
        frame "Finish Scenario 4 (Amplitude Sweep)" {
          n87 = Unbundle By Name(w577) -> ("f (Hz)"=w576:dbl, "Number of steps"=w574:i32, "Total time (s)"=w573:dbl, "amp_start (V)"=w571:dbl, "Modulation Depth (0.0 %)"=w563:dbl, "Channel (1:Channel 1)"=w572:i32, "amp_end (V)"=w570:dbl, "fc (Hz)"=w575:dbl, "DC Offset (V)"=w565:dbl)
          n88 = Build Array (concatenate)(w579, w569, w564, w568, w567, w576, w576, w575, w575, w574, w573, w563, w563, w572, w571, w570, w565) -> (w578:dbl[])
        }
        frame "Finish Cool Off Scenario 4 (Amplitude Sweep)" {
          n89 = Unbundle By Name(w594) -> ("f (Hz)"=w593:dbl, "Number of steps"=w591:i32, "Total time (s)"=w590:dbl, "amp_start (V)"=w588:dbl, "Modulation Depth (0.0 %)"=w580:dbl, "Channel (1:Channel 1)"=w589:i32, "amp_end (V)"=w587:dbl, "fc (Hz)"=w592:dbl, "DC Offset (V)"=w582:dbl)
          n90 = Build Array (concatenate)(w596, w586, w581, w585, w584, w593, w593, w592, w592, w591, w590, w580, w580, w589, w588, w587, w582) -> (w595:dbl[])
        }
        frame "Start Cool Off Scenario 4 (Amplitude Sweep)" {
          n91 = Unbundle By Name(w611) -> ("f (Hz)"=w610:dbl, "Number of steps"=w608:i32, "Total time (s)"=w607:dbl, "amp_start (V)"=w605:dbl, "Modulation Depth (0.0 %)"=w597:dbl, "Channel (1:Channel 1)"=w606:i32, "amp_end (V)"=w604:dbl, "fc (Hz)"=w609:dbl, "DC Offset (V)"=w599:dbl)
          n92 = Build Array (concatenate)(w613, w603, w598, w602, w601, w610, w610, w609, w609, w608, w607, w597, w597, w606, w605, w604, w599) -> (w612:dbl[])
        }
        frame "Threshold is gone while Scenario 4 (Amplitude Sweep)" {
          n93 = Unbundle By Name(w628) -> ("f (Hz)"=w627:dbl, "Number of steps"=w625:i32, "Total time (s)"=w624:dbl, "amp_start (V)"=w622:dbl, "Modulation Depth (0.0 %)"=w614:dbl, "Channel (1:Channel 1)"=w623:i32, "amp_end (V)"=w621:dbl, "fc (Hz)"=w626:dbl, "DC Offset (V)"=w616:dbl)
          n94 = Build Array (concatenate)(w630, w620, w615, w619, w618, w627, w627, w626, w626, w625, w624, w614, w614, w623, w622, w621, w616) -> (w629:dbl[])
        }
        frame "Start Depth Sweep" {
          w641 = 0
          n95 = Unbundle By Name(w640) -> ("f (Hz)"=w639:dbl, "Number of steps"=w638:i32, "Total time (s)"=w637:dbl, "Amplitude (V)"=w636:dbl, "depth_start (0.0 %)"=w635:dbl, "Channel (1:Channel 1)"=w633:i32, "fc (Hz)"=w632:dbl, "DC Offset (V)"=w631:dbl, "depth_end (0.0 %)"=w634:dbl)
          n96 = Build Array (concatenate)(w644, w641, w641, w641, w641, w639, w639, w632, w632, w638, w637, w635, w634, w633, w636, w636, w631) -> (w643:dbl[])
        }
        frame "Start Depth Sweep-smooth" {
          w655 = 0
          n97 = Unbundle By Name(w654) -> ("f (Hz)"=w653:dbl, "Number of steps"=w652:i32, "Total time (s)"=w651:dbl, "Amplitude (V)"=w650:dbl, "depth_start (0.0 %)"=w649:dbl, "Channel (1:Channel 1)"=w647:i32, "fc (Hz)"=w646:dbl, "DC Offset (V)"=w645:dbl, "depth_end (0.0 %)"=w648:dbl)
          n98 = Build Array (concatenate)(w658, w655, w655, w655, w655, w653, w653, w646, w646, w652, w651, w649, w648, w647, w650, w650, w645) -> (w657:dbl[])
        }
        frame "Finish Depth Sweep" {
          w669 = 0
          n99 = Unbundle By Name(w668) -> ("f (Hz)"=w667:dbl, "Number of steps"=w666:i32, "Total time (s)"=w665:dbl, "Amplitude (V)"=w664:dbl, "depth_start (0.0 %)"=w663:dbl, "Channel (1:Channel 1)"=w661:i32, "fc (Hz)"=w660:dbl, "DC Offset (V)"=w659:dbl, "depth_end (0.0 %)"=w662:dbl)
          n100 = Build Array (concatenate)(w672, w669, w669, w669, w669, w667, w667, w660, w660, w666, w665, w663, w662, w661, w664, w664, w659) -> (w671:dbl[])
        }
        frame "Finish Depth Sweep-smooth" {
          w683 = 0
          n101 = Unbundle By Name(w682) -> ("f (Hz)"=w681:dbl, "Number of steps"=w680:i32, "Total time (s)"=w679:dbl, "Amplitude (V)"=w678:dbl, "depth_start (0.0 %)"=w677:dbl, "Channel (1:Channel 1)"=w675:i32, "fc (Hz)"=w674:dbl, "DC Offset (V)"=w673:dbl, "depth_end (0.0 %)"=w676:dbl)
          n102 = Build Array (concatenate)(w686, w683, w683, w683, w683, w681, w681, w674, w674, w680, w679, w677, w676, w675, w678, w678, w673) -> (w685:dbl[])
        }
        frame "Depth Sweep Parameters Change" {
          w697 = 0
          n103 = Unbundle By Name(w696) -> ("f (Hz)"=w695:dbl, "Number of steps"=w694:i32, "Total time (s)"=w693:dbl, "Amplitude (V)"=w692:dbl, "depth_start (0.0 %)"=w691:dbl, "Channel (1:Channel 1)"=w689:i32, "fc (Hz)"=w688:dbl, "DC Offset (V)"=w687:dbl, "depth_end (0.0 %)"=w690:dbl)
          n104 = Build Array (concatenate)(w700, w697, w697, w697, w697, w695, w695, w688, w688, w694, w693, w691, w690, w689, w692, w692, w687) -> (w699:dbl[])
        }
        frame "Start Scenario 5 (Depth Sweep)" {
          n105 = Unbundle By Name(w714) -> ("f (Hz)"=w713:dbl, "Number of steps"=w712:i32, "Total time (s)"=w711:dbl, "Amplitude (V)"=w710:dbl, "depth_start (0.0 %)"=w709:dbl, "Channel (1:Channel 1)"=w707:i32, "fc (Hz)"=w706:dbl, "DC Offset (V)"=w705:dbl, "depth_end (0.0 %)"=w708:dbl)
          n106 = Build Array (concatenate)(w717, w701, w702, w703, w704, w713, w713, w706, w706, w712, w711, w709, w708, w707, w710, w710, w705) -> (w716:dbl[])
        }
        frame "Finish Scenario 5 (Depth Sweep)" {
          n107 = Unbundle By Name(w731) -> ("f (Hz)"=w730:dbl, "Number of steps"=w729:i32, "Total time (s)"=w728:dbl, "Amplitude (V)"=w727:dbl, "depth_start (0.0 %)"=w726:dbl, "Channel (1:Channel 1)"=w724:i32, "fc (Hz)"=w723:dbl, "DC Offset (V)"=w722:dbl, "depth_end (0.0 %)"=w725:dbl)
          n108 = Build Array (concatenate)(w734, w718, w719, w720, w721, w730, w730, w723, w723, w729, w728, w726, w725, w724, w727, w727, w722) -> (w733:dbl[])
        }
        frame "Start Cool Off Scenario 5 (Depth Sweep)" {
          n109 = Unbundle By Name(w748) -> ("f (Hz)"=w747:dbl, "Number of steps"=w746:i32, "Total time (s)"=w745:dbl, "Amplitude (V)"=w744:dbl, "depth_start (0.0 %)"=w743:dbl, "Channel (1:Channel 1)"=w741:i32, "fc (Hz)"=w740:dbl, "DC Offset (V)"=w739:dbl, "depth_end (0.0 %)"=w742:dbl)
          n110 = Build Array (concatenate)(w751, w735, w736, w737, w738, w747, w747, w740, w740, w746, w745, w743, w742, w741, w744, w744, w739) -> (w750:dbl[])
        }
        frame "Finish Cool Off Scenario 5 (Depth Sweep)" {
          n111 = Unbundle By Name(w765) -> ("f (Hz)"=w764:dbl, "Number of steps"=w763:i32, "Total time (s)"=w762:dbl, "Amplitude (V)"=w761:dbl, "depth_start (0.0 %)"=w760:dbl, "Channel (1:Channel 1)"=w758:i32, "fc (Hz)"=w757:dbl, "DC Offset (V)"=w756:dbl, "depth_end (0.0 %)"=w759:dbl)
          n112 = Build Array (concatenate)(w768, w752, w753, w754, w755, w764, w764, w757, w757, w763, w762, w760, w759, w758, w761, w761, w756) -> (w767:dbl[])
        }
        frame "Threshold is gone while Scenario 5 (Depth Sweep)" {
          n113 = Unbundle By Name(w782) -> ("f (Hz)"=w781:dbl, "Number of steps"=w780:i32, "Total time (s)"=w779:dbl, "Amplitude (V)"=w778:dbl, "depth_start (0.0 %)"=w777:dbl, "Channel (1:Channel 1)"=w775:i32, "fc (Hz)"=w774:dbl, "DC Offset (V)"=w773:dbl, "depth_end (0.0 %)"=w776:dbl)
          n114 = Build Array (concatenate)(w785, w769, w770, w771, w772, w781, w781, w774, w774, w780, w779, w777, w776, w775, w778, w778, w773) -> (w784:dbl[])
        }
      }
      n115 = for {
        tunnel: w22 -> [w793] mode=indexing
        shift-right: [w795] -> w14
        shift-left: w27 -> [w794]
        n116 = Format Value(format string="%.1f", value (0)=w793) -> (output string=w792:string)  [unwired: 1 in]
        n117 = Insert Into Array "Insert Into Array"(array=w794, new element=w792) -> (w795:string[])  [unwired: 1 in]
      }
      "Array" <- w14
      n118 = Insert Into Array(array=w14, new element=w12) -> (w13:string[])  [unwired: 1 in]
      n119 = Unbundle By Name("File Parameters") -> ("Path"=w54:path, "Recording Name"=w57:string)
      n120 = Path To String(path=w54) -> (string=w55:string)
      n121 = Concatenate Strings(w55, "\\", w57, "_logfile.csv") -> (w56:string)
      "output filename" <- w56
      n122 = String To Path(string=w56) -> (path=w51:path)
      n123 = call-poly <vilib>:"Write Delimited Spreadsheet.vi"("file path (dialog if empty)"=w51, "format (%s)"="%s", "1D data"=w13, "append to file? (new file:F)"=TRUE, "error in (no error)"=w58, "delimiter (\\t)"=";" ("delimiter (\\t)")) -> ("error out"=w47:errorcluster)  [unwired: 8 in, 1 out]
    }
  }
  "error out" <- w1
